vi "Create New Page.vi"(7 "Update Current Page (F)":bool, 8 "error in (no error)":errorcluster {"code" format="Error %.0f"}, 10 "Name":string, 11 "VIDoc Printer - Confluence In":refnum<class "VIDoc Printer - Confluence.lvclass">) -> (0 "error out":errorcluster {"code" format="Error %.0f"}, 1 "Created Page Info":T1, 2 "New Page Title":string, 3 "VIDoc Printer - Confluence Out":refnum<class "VIDoc Printer - Confluence.lvclass">)   [LabVIEW 2023, in "VIDoc Printer - Confluence.lvlib" / "VIDoc Printer - Confluence.lvclass"]
uses:
  VIDoc Printer - Confluence.lvclass
  Types/Page Info.ctl
  <userlib>/_PetranWay/LabVIEW Confluence API/Source/Confluence/Page/Page.lvclass
  VIDoc Printer - Confluence.lvclass/VIDoc Printer - Confluence.ctl
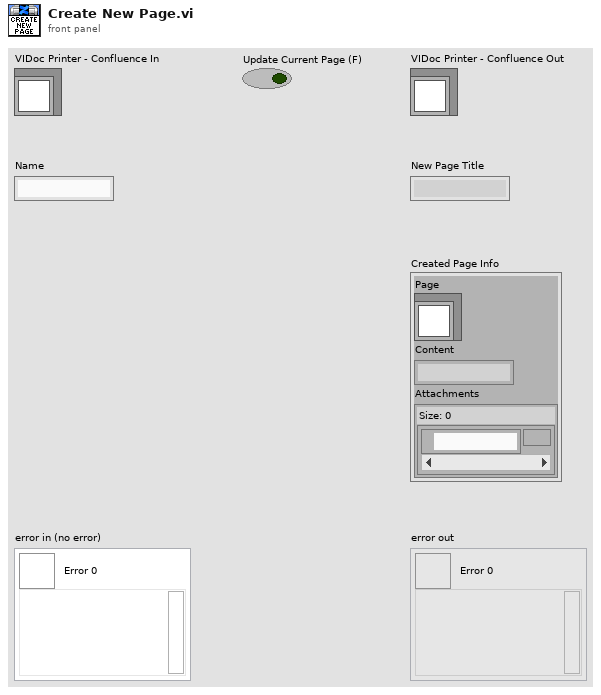
[diagram p1: front panel]
types:
  T1 = typedef "VIDoc Printer - Confluence.lvlib/VIDoc Printer - Confluence.lvclass/Page Info.ctl" = cluster{"Page":refnum<class "Page.lvclass">, "Content":string, "Attachments":set{path}}
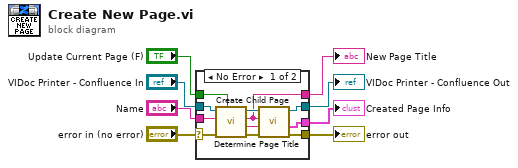
[diagram p0: block diagram]
diagram:
  n1 = case shown="No Error" "error in (no error)" {
    selector: "error in (no error)" -> [w14 w21]
    tunnel: [w13 w21] -> w7
    tunnel: [w16 w20] -> w5
    tunnel: "VIDoc Printer - Confluence In" -> [w15 w20]
    tunnel: "Name" -> [w12 _]
    tunnel: "Update Current Page (F)" -> [w11 _]
    tunnel: [w10 _] -> w2
    tunnel: [w9 _] -> w1
    frame No Error {
      n2 = call "Determine Page Title.vi"("Update Current Page (F)"=w11, "error in (no error)"=w14, "Name"=w12, "VIDoc Printer - Confluence In"=w15) -> ("error out"=w19:errorcluster, "Parent Page Title"=w18:string, "Page Title"=w9:string, "VIDoc Printer - Confluence Out"=w17:refnum<class "VIDoc Printer - Confluence.lvclass">)  [unwired: 4 in]
      n3 = call "Create Child Page.vi"("error in (no error)"=w19, "Parent Page Title"=w18, "New Page Title"=w9, "VIDoc Printer - Confluence In"=w17) -> ("error out"=w13:errorcluster, "Created Page Info"=w10:T1, "VIDoc Printer - Confluence Out"=w16:refnum<class "VIDoc Printer - Confluence.lvclass">)  [unwired: 5 in]
    }
    frame Error {
    }
  }
  "error out" <- w7
  "VIDoc Printer - Confluence Out" <- w5
  "Created Page Info" <- w2
  "New Page Title" <- w1
